vi "Handle Errors.vi"(8 "error in (no error)":errorcluster, 10 "Location":string, 11 "Process In":refnum<class "Process.lvclass">) -> (0 "error out":errorcluster, 3 "Process Out":refnum<class "Process.lvclass">)   [LabVIEW 2020, in "Process.lvclass"]
doc: "Delegates any error to the Error Handler Interface configured using the Set Error Handler.vi method. This method is used by the framework in the process loop, but may also be used to send errors that cannot be handled locally to the centralized error handler."
uses:
  Process.lvclass
  Error Handler Interface/Error Handler Interface.lvclass
  Process.lvclass/Process.ctl
  Lifecycle/Get Lifecycle State.vi
  <vilib>/Utility/error.llb/Error Cluster From Error Code.vi
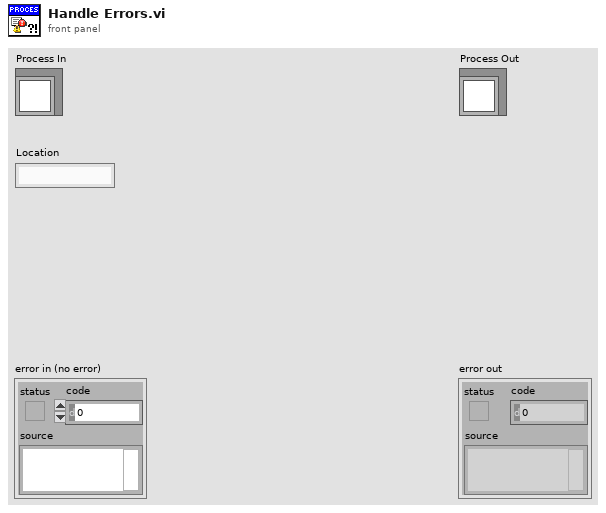
[diagram p1: front panel]
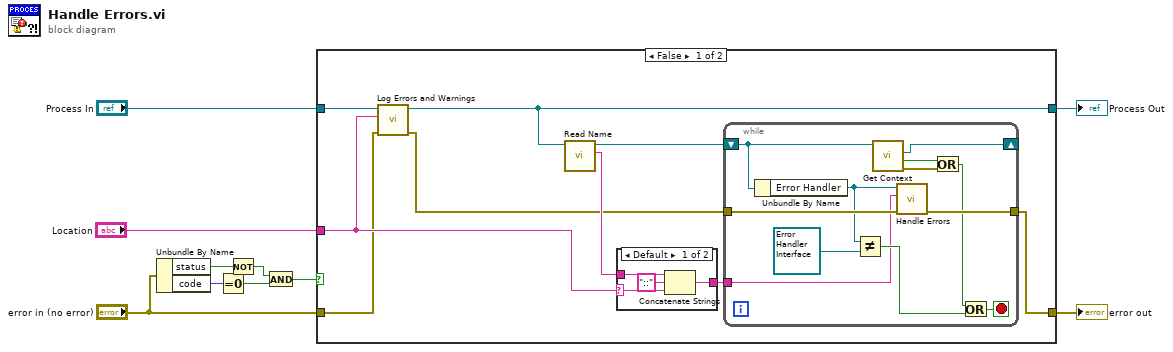
[diagram p0: block diagram]
diagram:
  n1 = Unbundle By Name("error in (no error)") -> ("status"=w2:bool, "code"=w5:i32)
  n2 = Equal To 0?(x=w5) -> (x = 0?=w4:bool)
  n3 = Not(x=w2) -> (.not. x?=w1:bool)
  n4 = And(x=w1, y=w4) -> (x .and. y?=w3:bool)
  n5 = case shown="False" w3 {
    tunnel: [w16 w37] -> w10
    tunnel: [w15 w38] -> w8
    tunnel: "Process In" -> [w14 w38]
    tunnel: "Location" -> [w13 _]
    tunnel: "error in (no error)" -> [w11 w37]
    frame False {
      n6 = call "Log Errors and Warnings.vi"("error in (no error)"=w11, "Location"=w13, "Process In"=w14) -> ("error out"=w12:errorcluster, "Process Out"=w15:refnum<class "Process.lvclass">)  [unwired: 7 in]
      n7 = call "Read Name.vi"("Process In"=w15) -> ("Qualified Name"=w19:string, "Process Out"=w18:refnum<class "Process.lvclass">)  [unwired: 7 in, 2 out]
      n8 = case shown="Default" w13 {
        selector: w13 -> [w33 _]
        tunnel: w19 -> [w35 w36]
        tunnel: [w34 w36] -> w17
        frame Default {
          n9 = Concatenate Strings(w35, "::" ("string"), w33) -> (w34:string)
        }
        frame "" {
        }
      }
      n10 = while {
        shift-right: [w26] -> _
        shift-left: w18 -> [w21]
        tunnel: w17 -> [w20]
        tunnel: w12 -> [w31]
        tunnel: [w30] -> w16
        stop <- w23 stop-if-true
        n11 = Unbundle By Name(w21) -> ("Error Handler"=w25:refnum<class "Error Handler Interface.lvclass">)
        n12 = Not Equal?(x=w25, y=refnum<class "Error Handler Interface.lvclass"> refnum ("Error Handler")) -> (x != y?=w22:bool)
        n13 = call "Get Context.vi"("Process In"=w21) -> ("error out"=w28:errorcluster, "Top Level?"=w29:bool, "Context"=w26:refnum<class "Process.lvclass">)  [unwired: 7 in, 1 out]
        n14 = call-dynamic "Handle Errors.vi"("error in (no error)"=w31, "Location"=w20, "Error Handler Interface In"=w25) -> ("error out"=w30:errorcluster)  [unwired: 7 in, 1 out]
        n15 = Or(x=w29, y=w28) -> (x .or. y?=w27:bool)
        n16 = Or(x=w27, y=w22) -> (x .or. y?=w23:bool)
      }
    }
    frame True {
    }
  }
  "error out" <- w10
  "Process Out" <- w8
